vi "XYGraph.vi"() -> ()   [LabVIEW 2024]
uses:
  <vilib>/Utility/miscctls.llb/LVBoundsTypeDef.ctl
  <vilib>/Utility/miscctls.llb/LVPositionTypeDef.ctl
  <vilib>/picture/picture.llb/imagedata.ctl
panel:
  out "XY Graph 3":cluster{i32[], i32[]}[](graph)
  out "subarray":i32[](array[numeric])
  out "XY Graph 2":cluster{i32[], i32[]}[](graph)
  out "Image Data":T1
  out "Position":T2
  out "Bounds":T3
  out "タブ数":i32
  in  "Tab Control":enum32{"Page 1", "Page 2"}(tab)
  out "XY Graph":cluster{i32[], i32[]}(graph)
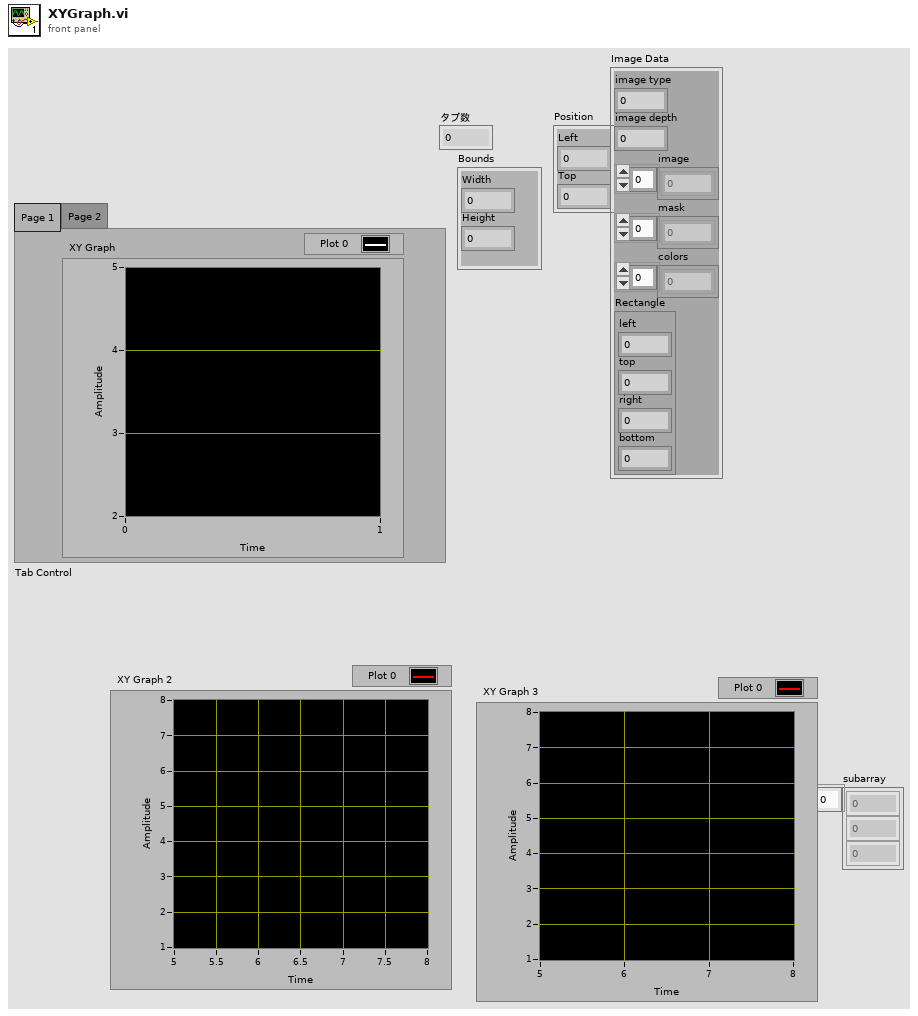
[diagram p1: front panel]
types:
  T1 = typedef "imagedata.ctl" = cluster{"image type":i32, "image depth":i32, "image":u8[], "mask":u8[], "colors":u32[], "Rectangle":cluster{"left":i16, "top":i16, "right":i16, "bottom":i16}}
  T2 = typedef "LVPositionTypeDef.ctl" = cluster{"Left":i32, "Top":i32}
  T3 = typedef "LVBoundsTypeDef.ctl" = cluster{"Width":u32, "Height":u32}
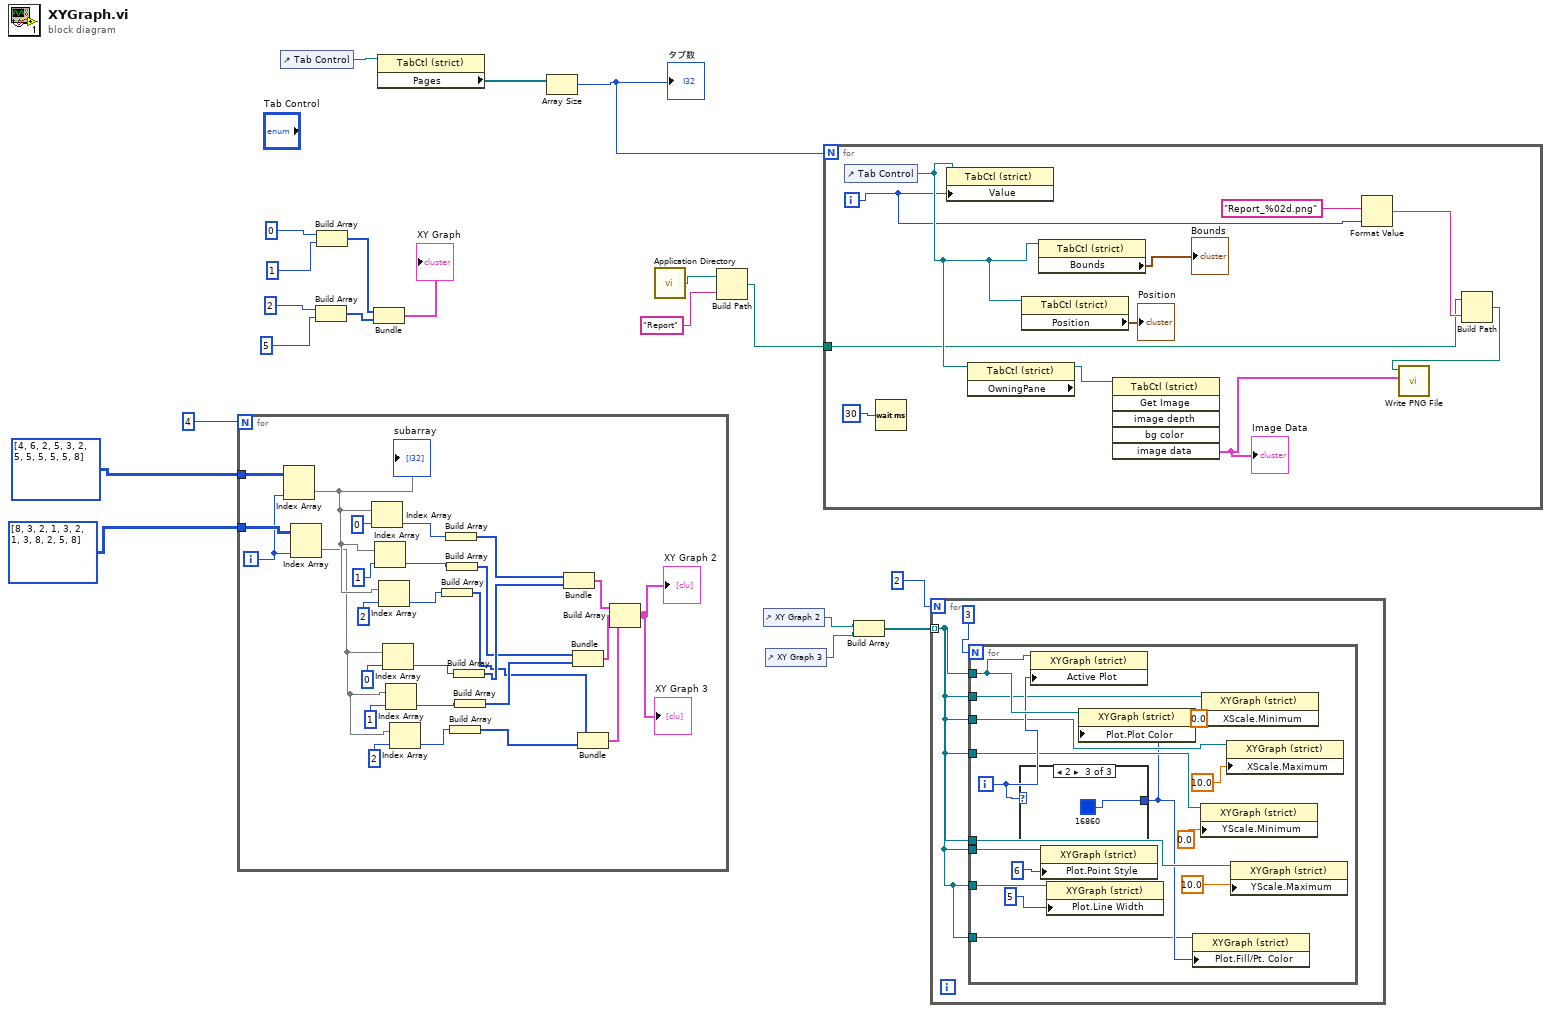
[diagram p0: block diagram]
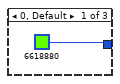
[diagram p2: hidden frame]
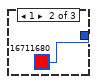
[diagram p3: hidden frame]
diagram:
  n1 = for {
    N: 4 -> [_]
    tunnel: i32[][] [[4, 6, 2, 5], [3, 2, 5, 5], [5, 5, 5, 8]] -> [w47]
    tunnel: i32[][] [[8, 3, 2, 1], [3, 2, 1, 3], [8, 2, 5, 8]] -> [w46]
    i -> [w45]
    n2 = Index Array(array=w47, index (col)=w45) -> (element=w41:i32[])  [unwired: 1 in]
    "subarray" <- w41
    n3 = Index Array(array=w46, index (col)=w45) -> (element=w37:i32[])  [unwired: 1 in]
    n4 = Index Array(array=w41, index=0) -> (element=w36:i32)
    n5 = Index Array(array=w41, index=1) -> (element=w35:i32)
    n6 = Index Array(array=w41, index=2) -> (element=w34:i32)
    n7 = Index Array(array=w37, index=0) -> (element=w33:i32)
    n8 = Index Array(array=w37, index=1) -> (element=w32:i32)
    n9 = Index Array(array=w37, index=2) -> (element=w31:i32)
    n10 = Build Array(w34) -> (w26:i32[])
    n11 = Build Array(w36) -> (w30:i32[])
    n12 = Build Array(w35) -> (w28:i32[])
    n13 = Build Array(w31) -> (w25:i32[])
    n14 = Build Array(w33) -> (w29:i32[])
    n15 = Build Array(w32) -> (w27:i32[])
    n16 = Bundle(w30, w29) -> (w24:cluster{i32[], i32[]})  [unwired: 1 in]
    n17 = Bundle(w28, w27) -> (w23:cluster{i32[], i32[]})  [unwired: 1 in]
    n18 = Bundle(w26, w25) -> (w22:cluster{i32[], i32[]})  [unwired: 1 in]
    n19 = Build Array(w24, w23, w22) -> (→"XY Graph 2" →"XY Graph 3":cluster{i32[], i32[]}[])
  }
  n20 = control-ref of="Tab Control"() -> (w13:refnum<vi>)
  n21 = Build Array(2, 5) -> (w15:i32[])
  n22 = Build Array(0, 1) -> (w16:i32[])
  n23 = Bundle(w16, w15) -> (→"XY Graph":cluster{i32[], i32[]})  [unwired: 1 in]
  n24 = property class="TabCtl (strict)"(reference=w13) -> ("Pages"=w12:refnum<vi>[])  [unwired: 1 in, 2 out]
  n25 = Array Size(array=w12) -> (size(s)=w11:i32)
  "タブ数" <- w11
  n26 = call <vilib>:"Application Directory.vi"() -> ("Application Directory"=w9:path)
  n27 = Build Path(base path=w9, name or relative path="Report") -> (appended path=w8:path)
  n28 = control-ref of="XY Graph 2"() -> (w4:refnum<vi>)
  n29 = control-ref of="XY Graph 3"() -> (w3:refnum<vi>)
  n30 = for {
    N: w11 -> [_]
    tunnel: w8 -> [w48]
    i -> [w50]
    n31 = control-ref of="Tab Control"() -> (w55:refnum<vi>)
    n32 = Wait (ms)(milliseconds to wait=30) -> ()  [unwired: 1 out]
    n33 = property class="TabCtl (strict)"(reference=w55, "Value"=w50) -> ()  [unwired: 1 in, 2 out]
    n34 = property class="TabCtl (strict)" props=["OwningPane"](reference=w55) -> (reference out=w54:refnum<vi>)  [unwired: 1 in, 2 out]
    n35 = property class="TabCtl (strict)"(reference=w55) -> ("Position"=→"Position":T2)  [unwired: 1 in, 2 out]
    n36 = property class="TabCtl (strict)"(reference=w55) -> ("Bounds"=→"Bounds":T3)  [unwired: 1 in, 2 out]
    n37 = invoke class="TabCtl (strict)" method="Get Image"(reference=w54) -> ("image data"=w53:T1)  [unwired: 5 in, 5 out]
    "Image Data" <- w53
    n38 = Format Value(format string="Report_%02d.png", value (0)=w50) -> (output string=w49:string)  [unwired: 1 in]
    n39 = Build Path(base path=w48, name or relative path=w49) -> (appended path=w52:path)
    n40 = call <vilib>:"Write PNG File.vi"("image data"=w53, "path to PNG file"=w52) -> ()  [unwired: 8 in, 2 out]
  }
  n41 = Build Array(w4, w3) -> (w2:refnum<vi>[])
  n42 = for {
    N: 2 -> [_]
    tunnel: w2 -> [w59] mode=indexing
    n43 = for {
      N: 3 -> [_]
      tunnel: w59 -> [w76]
      tunnel: w59 -> [w74]
      tunnel: w59 -> [w73]
      tunnel: w59 -> [w70]
      tunnel: w59 -> [w68]
      tunnel: w59 -> [w66]
      tunnel: w59 -> [w64]
      tunnel: w59 -> [w61]
      i -> [w75]
      n44 = case shown="2" w75 {
        tunnel: [u32 6618880 ("Plot.Plot Color") u32 16711680 ("Plot.Plot Color") u32 16860 ("Plot.Plot Color")] -> w62
        frame 0, Default {
        }
        frame 1 {
        }
        frame 2 {
        }
      }
      n45 = property class="XYGraph (strict)"(reference=w76, "Active Plot"=w75) -> ()  [unwired: 1 in, 2 out]
      n46 = property class="XYGraph (strict)"(reference=w74, "Plot.Point Style"=u8 6) -> ()  [unwired: 1 in, 2 out]
      n47 = property class="XYGraph (strict)"(reference=w73, "Plot.Line Width"=u8 5) -> ()  [unwired: 1 in, 2 out]
      n48 = property class="XYGraph (strict)"(reference=w76, "Plot.Plot Color"=w62) -> ()  [unwired: 1 in, 2 out]
      n49 = property class="XYGraph (strict)"(reference=w61, "Plot.Fill/Pt. Color"=w62) -> ()  [unwired: 1 in, 2 out]
      n50 = property class="XYGraph (strict)"(reference=w66, "YScale.Minimum"=0.0 ("Y Scale.Range:Minimum")) -> ()  [unwired: 1 in, 2 out]
      n51 = property class="XYGraph (strict)"(reference=w70, "XScale.Minimum"=0.0 ("X Scale.Range:Minimum")) -> ()  [unwired: 1 in, 2 out]
      n52 = property class="XYGraph (strict)"(reference=w64, "XScale.Maximum"=10.0 ("X Scale.Range:Maximum")) -> ()  [unwired: 1 in, 2 out]
      n53 = property class="XYGraph (strict)"(reference=w68, "YScale.Maximum"=10.0 ("Y Scale.Range:Maximum")) -> ()  [unwired: 1 in, 2 out]
    }
  }
